vi "Hello GDEVCON!.vi"() -> ()   [LabVIEW 2026]
uses:
  <vilib>/addons/_TSC/TSC Pop-Up/Popup/message info--typedef.ctl
  <vilib>/addons/_TSC/TSC Pop-Up/Theme/Theme.lvclass
  <vilib>/addons/_TSC/TSC Pop-Up/Custom/Custom - One Button/Custom - One Button.lvclass
  <vilib>/addons/_TSC/TSC Pop-Up/Popup/Popup.lvclass
panel:
  out "Error Out":errorcluster
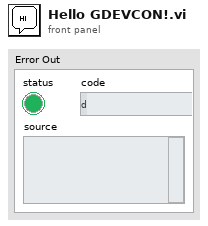
[diagram p1: front panel]
types:
  T1 = typedef "Pop-Up.lvlib/Popup.lvclass/message info--typedef.ctl" = cluster{"Message Height":i32, "Message Width":i32, "Message Location":enum16{"Top", "Bottom", "Right", "Left"}}
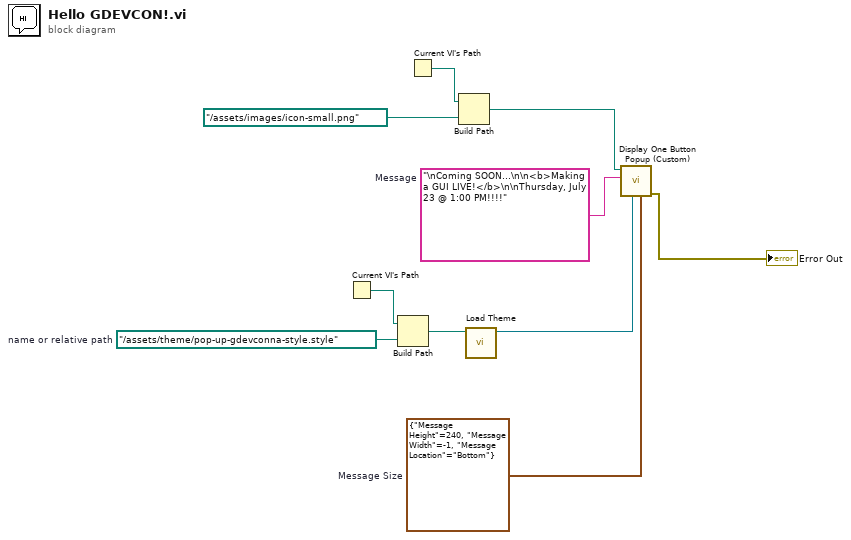
[diagram p0: block diagram]
diagram:
  w1 = T1 {"Message Height"=240, "Message Width"=-1, "Message Location"=enum."Bottom"}  # Message Size
  w7 = path "../assets/theme/pop-up-gdevconna-style.style"  # name or relative path
  w9 = "\nComing SOON...\n\n<b>Making a GUI LIVE!</b>\n\nThursday, July 23 @ 1:00 PM!!!!"  # Message
  n1 = Current VI's Path() -> (path=w8:path)
  n2 = Build Path(base path=w8, name or relative path=w7) -> (appended path=w6:path)
  n3 = Current VI's Path() -> (path=w3:path)
  n4 = Build Path(base path=w3, name or relative path=path "../assets/images/icon-small.png") -> (appended path=w2:path)
  n5 = call <vilib>:"Load Theme.vi"("File Path"=w6) -> ("Theme"=w5:refnum<class "Theme.lvclass">)  [unwired: 9 in, 1 out]
  n6 = call <vilib>:"Display One Button Popup (Custom).vi"("Message Size"=w1, "Theme"=w5, "Message"=w9, "Graphic"=w2) -> ("Error Out"=→"Error Out":errorcluster)  [unwired: 7 in]
